vi "setDACjob.vi"(4 "blue":dbl[](array[numeric]), 5 "red":dbl[](array[numeric]), 6 "sample sn":string[](array[string]), 7 "sample port":refnum<visa-resource-name>[](array[refnum])) -> (0 "error":errorcluster[](array[cluster]), 1 "Array":bool[](array[boolean]))   [LabVIEW 2012]
uses:
  globalstatus.vi
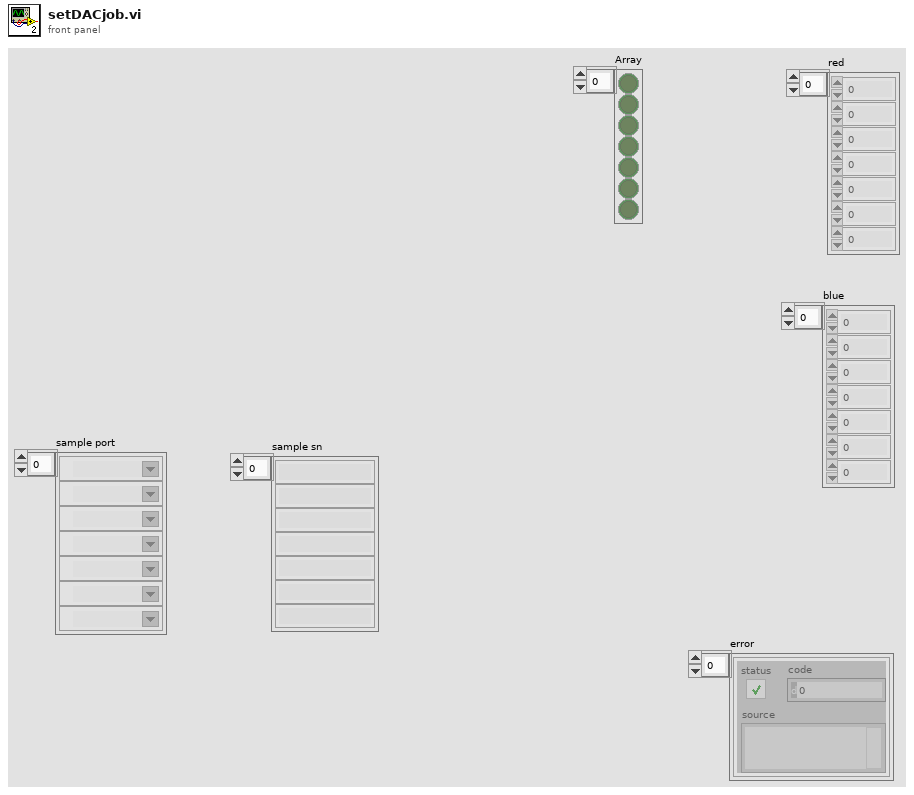
[diagram p1: front panel]
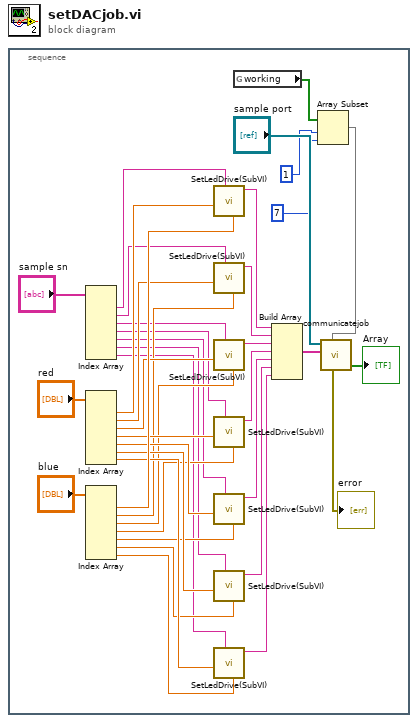
[diagram p0: block diagram]
diagram:
  n1 = stacked-sequence {
    frame #0 {
      n2 = Index Array(array="sample sn") -> (element #1=w22:string, element #2=w21:string, element #3=w20:string, element #4=w19:string, element #5=w18:string, element #6=w17:string, element #7=w16:string)  [unwired: 7 in]
      n3 = Index Array(array="red") -> (element #1=w37:dbl, element #2=w35:dbl, element #3=w34:dbl, element #4=w33:dbl, element #5=w32:dbl, element #6=w31:dbl, element #7=w30:dbl)  [unwired: 7 in]
      n4 = Index Array(array="blue") -> (element #1=w36:dbl, element #2=w29:dbl, element #3=w28:dbl, element #4=w27:dbl, element #5=w26:dbl, element #6=w25:dbl, element #7=w24:dbl)  [unwired: 7 in]
      n5 = call "SetLedDrive(SubVI).vi"("blue dac"=w36, "sn"=w22, "red dac"=w37) -> ("String"=w14:string)  [unwired: 8 in]
      n6 = call "SetLedDrive(SubVI).vi"("blue dac"=w29, "sn"=w21, "red dac"=w35) -> ("String"=w13:string)  [unwired: 8 in]
      n7 = call "SetLedDrive(SubVI).vi"("blue dac"=w28, "sn"=w20, "red dac"=w34) -> ("String"=w12:string)  [unwired: 8 in]
      n8 = call "SetLedDrive(SubVI).vi"("blue dac"=w27, "sn"=w19, "red dac"=w33) -> ("String"=w11:string)  [unwired: 8 in]
      n9 = call "SetLedDrive(SubVI).vi"("blue dac"=w26, "sn"=w18, "red dac"=w32) -> ("String"=w10:string)  [unwired: 8 in]
      n10 = call "SetLedDrive(SubVI).vi"("blue dac"=w25, "sn"=w17, "red dac"=w31) -> ("String"=w9:string)  [unwired: 8 in]
      n11 = call "SetLedDrive(SubVI).vi"("blue dac"=w24, "sn"=w16, "red dac"=w30) -> ("String"=w8:string)  [unwired: 8 in]
      n12 = global read "globalstatus.vi" "working"() -> (w3:bool[])
      n13 = Build Array(w14, w13, w12, w11, w10, w9, w8) -> (w7:string[])
      n14 = Array Subset(array=w3, index=1, length=7) -> (w4:bool[])
      n15 = call "communicatejob.vi"("sample port"="sample port", "condition"=w4, "send command"=w7) -> ("error"=→"error":errorcluster[], "receive result"=→"Array":bool[])  [unwired: 2 in, 2 out]
    }
  }
